vi "uService GUI.vi"(8 "error in (no error)":errorcluster, 11 "uService Template in":refnum<class "Dummy.lvclass">) -> (3 "uService Template out":refnum<class "Dummy.lvclass">)   [LabVIEW 2020, in "Dummy.lvlib" / "Dummy.lvclass"]
uses:
  Dummy.lvclass
  TALOS/TALOS_PPL.lvlibp/Father of all uServices/Father of all uServices/Father of all uServices.lvclass
  C:/LabVIEW Code/aegis-labview-code/TALOS/TALOS_PPL.lvlibp/Father of all uServices/Father of all uServices/Father of all uServices.lvclass
panel:
  in  "Test":bool
  out "LED":bool
  out "RUN":bool
  in  "stop New uService":bool
  in  "Toggle LED":bool
  # "Dummy!"
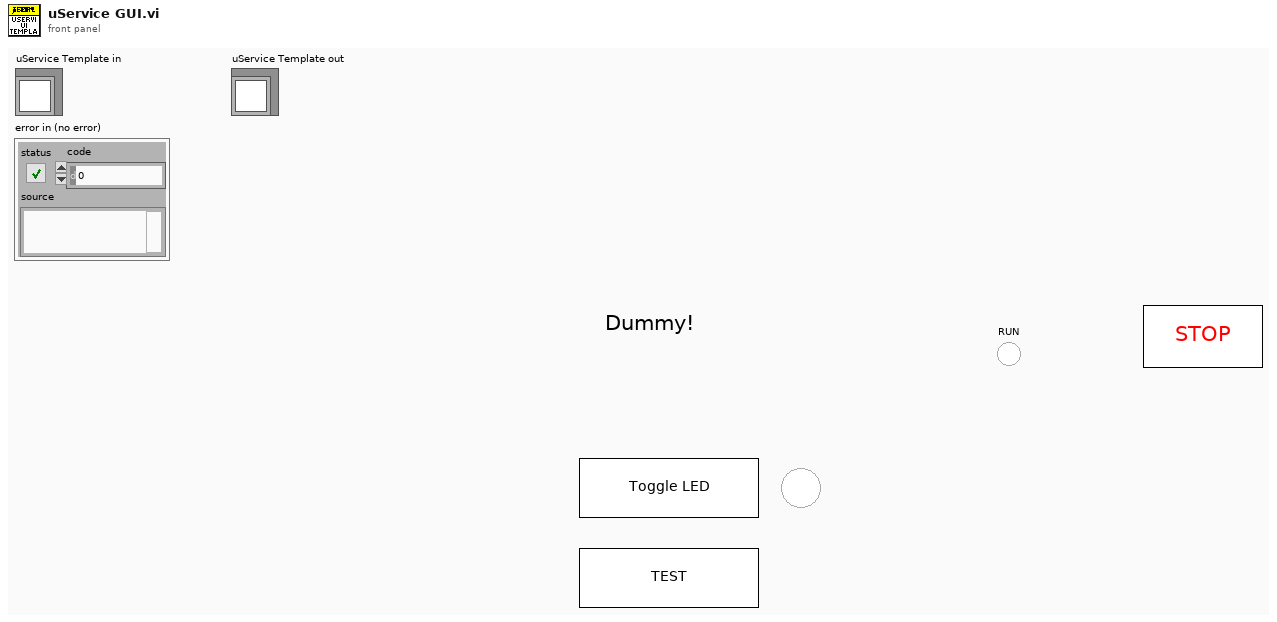
[diagram p1: front panel]
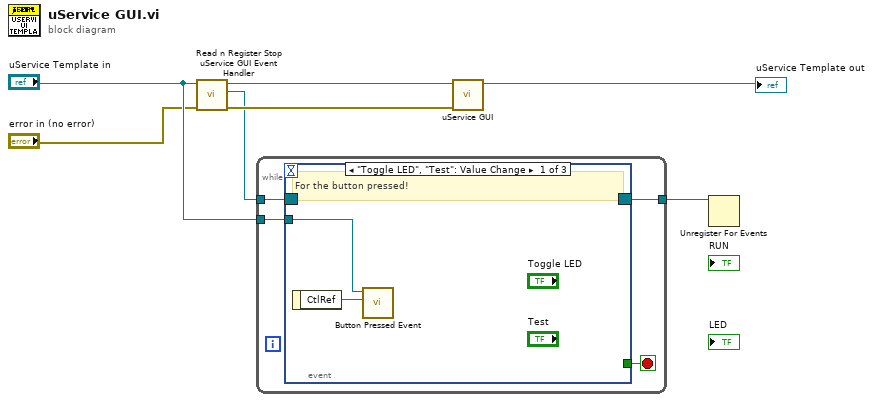
[diagram p0: block diagram]
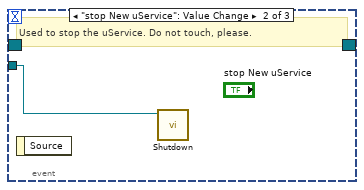
[diagram p2: hidden frame]
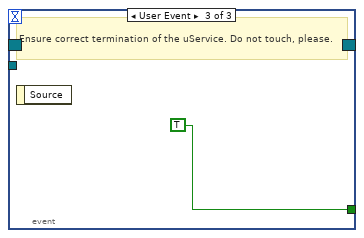
[diagram p3: hidden frame]
diagram:
  n1 = call-dynamic "Read n Register Stop uService GUI Event Handler .vi"("error in (no error)"="error in (no error)", "uService Template in"="uService Template in") -> ("error out"=w5:errorcluster, "Stop uService GUI Event Ref"=w4:refnum<event-registration>, "uService Template out"=w6:refnum<class "Dummy.lvclass">)  [unwired: 7 in]
  n2 = while {
    tunnel: [w11] -> w7
    tunnel: w4 -> [w9]
    tunnel: "uService Template in" -> [w8]
    stop <- w10 stop-if-true
    n3 = event shown="[0] \"Toggle LED\", \"Test\": Value Change" {
      selector: w9 -> [_ _ _]
      dyn-events: [_ _ _] -> w11
      timeout: _ -> [_ _ _]
      tunnel: [_ _ TRUE] -> w10
      tunnel: w8 -> [w13 w14 _]
      event "Toggle LED", "Test": Value Change {
        # "For the button pressed!"
        n4 = event-data() -> ("CtlRef"=w12:refnum<vi>)  [unwired: 1 in]
        n5 = call-dynamic "Button Pressed Event.vi"("CtlRef"=w12, "uService Template in"=w13) -> ()  [unwired: 8 in, 2 out]
      }
      event "stop New uService": Value Change {
        # "Used to stop the uService. Do not touch, please."
        n6 = event-data() -> ()  [unwired: 1 in, 1 out]
        n7 = call "Shutdown.vi"("Father of all uServices in"=w14) -> ()  [unwired: 9 in, 2 out]
      }
      event User Event {
        # "Ensure correct termination of the uService. Do not touch, please."
        n8 = event-data() -> ()  [unwired: 1 in, 1 out]
      }
    }
  }
  n9 = call-parent "uService GUI.vi"("error in (no error)"=w5, "uService Template in"=w6) -> ("uService Template out"=→"uService Template out":refnum<class "Dummy.lvclass">)  [unwired: 9 in]
  n10 = Unregister For Events(event registration refnum=w7) -> ()  [unwired: 1 in, 1 out]
